vi "Feu.vi"() -> ()   [LabVIEW 2018]
panel:
  in  "stop":bool
  in  "Phase 4":i16
  in  "Phase 3":i16
  in  "Phase 2":i16
  in  "Phase 1":i16
  out "Vert":bool
  out "Orange":bool
  out "Rouge":bool
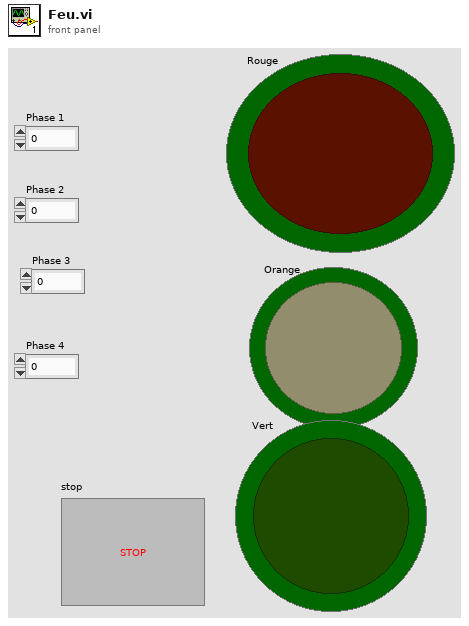
[diagram p1: front panel]
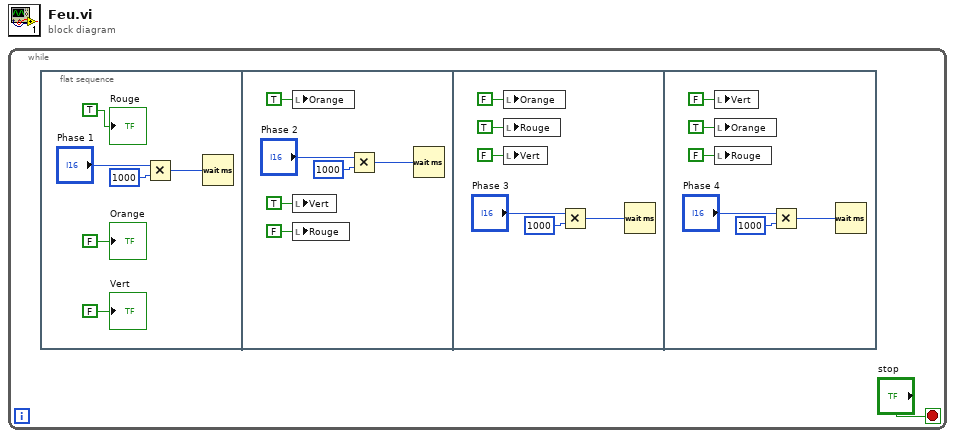
[diagram p0: block diagram]
diagram:
  n1 = while {
    stop <- "stop" stop-if-true
    n2 = flat-sequence {
      frame #0 {
        n3 = Multiply(x="Phase 1", y=i16 1000) -> (x*y=w2:i16)
        n4 = Wait (ms)(milliseconds to wait=w2) -> ()  [unwired: 1 out]
        "Rouge" <- TRUE ("Boolean")
        "Orange" <- FALSE ("Boolean 2")
        "Vert" <- FALSE ("Boolean 3")
      }
      frame #1 {
        n5 = local write "Orange"(TRUE ("Boolean 2")) -> ()
        n6 = local write "Vert"(TRUE ("Boolean 3")) -> ()
        n7 = local write "Rouge"(FALSE ("Boolean")) -> ()
        n8 = Multiply(x="Phase 2", y=i16 1000) -> (x*y=w8:i16)
        n9 = Wait (ms)(milliseconds to wait=w8) -> ()  [unwired: 1 out]
      }
      frame #2 {
        n10 = local write "Orange"(FALSE ("Boolean 2")) -> ()
        n11 = local write "Rouge"(TRUE ("Boolean")) -> ()
        n12 = local write "Vert"(FALSE ("Boolean 3")) -> ()
        n13 = Multiply(x="Phase 3", y=i16 1000) -> (x*y=w14:i16)
        n14 = Wait (ms)(milliseconds to wait=w14) -> ()  [unwired: 1 out]
      }
      frame #3 {
        n15 = local write "Vert"(FALSE ("Boolean 3")) -> ()
        n16 = local write "Orange"(TRUE ("Boolean 2")) -> ()
        n17 = local write "Rouge"(FALSE ("Boolean")) -> ()
        n18 = Multiply(x="Phase 4", y=i16 1000) -> (x*y=w20:i16)
        n19 = Wait (ms)(milliseconds to wait=w20) -> ()  [unwired: 1 out]
      }
    }
  }
